vi "cat binary to string.vi"(10 "String in":string, 11 "ETX":i32) -> (3 "String out":string)   [LabVIEW 2016]
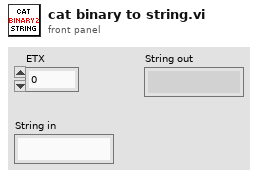
[diagram p1: front panel]
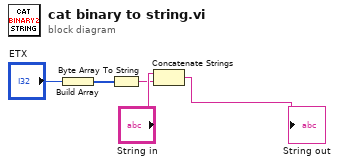
[diagram p0: block diagram]
diagram:
  n1 = Build Array("ETX") -> (w1:i32[])
  n2 = Byte Array To String(unsigned byte array=w1) -> (string=w2:string)
  n3 = Concatenate Strings("String in", w2) -> (→"String out":string)
